vi "Seleccionar.vi"(8 "error in (no error)":errorcluster, 10 "Productos":i32(listbox), 11 "Soda Actor in":refnum<class "Soda Actor.lvclass">) -> (0 "error out":errorcluster, 3 "Soda Actor out":refnum<class "Soda Actor.lvclass">)   [LabVIEW 2019, in "Soda Actor.lvlib" / "Soda Actor.lvclass"]
uses:
  Soda Actor.lvclass
  C:/Program Files (x86)/National Instruments/LabVIEW 2019/vi.lib/ActorFramework/Actor/Actor.lvclass
  <vilib>/ActorFramework/Actor/Actor.lvclass/Actor.ctl
  Soda Actor.lvclass/Soda Actor.ctl
  UI Actor Messages/seleccion Msg/seleccion Msg.lvclass/seleccion Msg.ctl
  <vilib>/ActorFramework/Message Enqueuer/Message Enqueuer.lvclass/Message Enqueuer.ctl
  <vilib>/ActorFramework/Message Enqueuer/Enqueue.vi
  UI Actor Messages/seleccion Msg/seleccion Msg.lvclass
  C:/Program Files (x86)/National Instruments/LabVIEW 2019/vi.lib/ActorFramework/Message/Message.lvclass
  <vilib>/ActorFramework/Message Priority Queue/Priority Enqueue.vi
  <vilib>/ActorFramework/Actor/Actor.lvclass
panel:
  in  "array":string[](array[string])
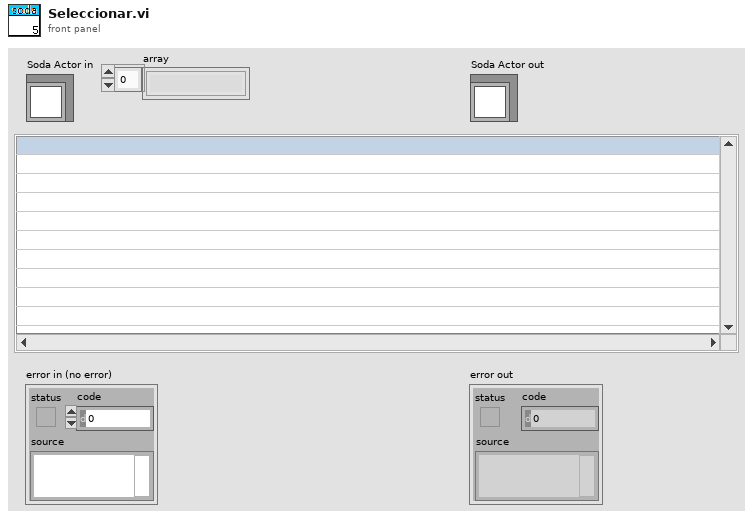
[diagram p1: front panel]
types:
  T1 = cluster{"array[0]":string, "array[1]":string, "array[2]":string, "array[3]":string, "array[4]":string, "array[5]":string, "array[6]":string, "array[7]":string, "array[8]":string}
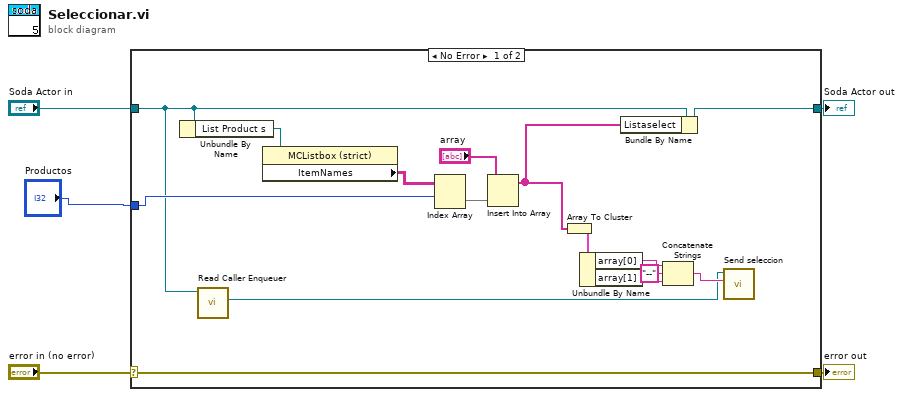
[diagram p0: block diagram]
diagram:
  n1 = case shown="No Error" "error in (no error)" {
    selector: "error in (no error)" -> [w20 w22]
    tunnel: [w20 w22] -> w4
    tunnel: [w15 w21] -> w2
    tunnel: "Soda Actor in" -> [w8 w21]
    tunnel: "Productos" -> [w9 _]
    frame No Error {
      n2 = Unbundle By Name(w8) -> ("List Product s"=w19:refnum<vi>)
      n3 = call <vilib>:"Read Caller Enqueuer.vi"("Actor"=w8) -> ("Caller Enqueuer"=w6:refnum<class "Message Enqueuer.lvclass">)  [unwired: 10 in]
      n4 = property class="MCListbox (strict)"(reference=w19) -> ("ItemNames"=w18:string[][])  [unwired: 1 in, 2 out]
      n5 = Index Array "Index Array"(array=w18, index (row)=w9) -> (element=w17:string[])  [unwired: 1 in]
      n6 = Insert Into Array "Insert Into Array"(array="array", new element=w17) -> (w14:string[])  [unwired: 1 in]
      n7 = Array To Cluster(array=w14) -> (cluster=w13:T1)
      n8 = Unbundle By Name(w13) -> ("array[0]"=w12:string, "array[1]"=w11:string)
      n9 = Bundle By Name(cluster=w8, "Listaselect"=w14) -> (w15:refnum<class "Soda Actor.lvclass">)
      n10 = Concatenate Strings(w12, "--" ("string"), w11) -> (w7:string)
      n11 = call "Send seleccion.vi"("Seleccion"=w7, "Message Enqueuer"=w6) -> ()  [unwired: 8 in, 2 out]
    }
    frame Error {
    }
  }
  "error out" <- w4
  "Soda Actor out" <- w2
